vi "SS2 Live_Create HDF5 File.vi"(8 "error in (no error)":errorcluster, 11 "Current Data Set":i32) -> (0 "Error Out":errorcluster, 1 "Notebook Message":string, 2 "# Image Sets":u32, 3 "# Data Sets":i32, 5 "Data Q Name":string)   [LabVIEW 2019]
uses:
  SS2 Live_Settings List.ctl
  SS2 Live_File Information.ctl
  SS2 DAQ Parameters 2.ctl
  SS2 Gate Definition.ctl
  <vilib>/addons/h5labview2/file/H5Fmode.ctl
  <vilib>/Utility/error.llb/Error Cluster From Error Code.vi
  <vilib>/ErrorRing/Error Ring.xnode
  <vilib>/addons/h5labview2/file/H5F.lvlib
panel:
  out "File Folder":path
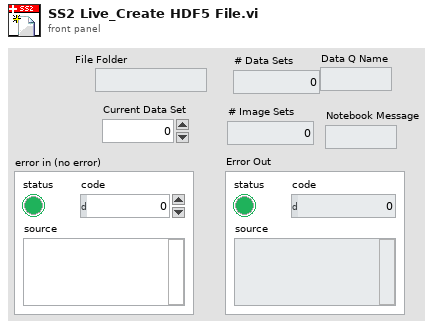
[diagram p1: front panel]
types:
  T1 = typedef "SS2 DAQ Parameters 2.ctl" = cluster{"10 bits":bool, "# Exposure Sequences":u32, "# 1-bit Frame per Gate":u32, "Gate Shift":u32, "# Gates per Set":u32, "# Sets":u32, "Laser Period":dbl[unit], "Gate Offset":u32, "Auto-adjust Gate Offset":bool, "Gate Definition":T2}
  T2 = typedef "SS2 Gate Definition.ctl" = cluster{"gs_psincdec_0":u32, "gs_psincdec_1":u32, "gs_psincdec_2":u32, "gs_psincdec_3":u32, "gs_no_shift_adj_1":u32, "gs_no_shift_adj_2":u32, "gs_no_shift_adj_3":u32}
  T3 = typedef "SS2 Live_Settings List.ctl" = enum16{"FPGA:Bitfile Path", "FPGA:Bitfile Version", "Acquisition Parameters:SS2 DAQ Parameters", "Acquisition Parameters:Gate Configuration Array", "Acquisition Parameters:Buffer Size (# Gates)", "File Information:File Information", "File Information:# Datasets in Series", "Image Parameters:Image ROI Information", "Image Parameters:Image Binning Options", "UI Parameters:Histogram Bins Number"}
  T4 = typedef "SS2 Live_File Information.ctl" = cluster{"File Folder":path, "File Name":string, "File Index":u32, "Author":string, "Sample":string, "Compression":bool}
  T5 = typedef "H5F.lvlib/H5Fmode.ctl" = enum16{"read-only", "read-write", "overwrite", "create new", "open or create"}
  T6 = typedef "hid_t.ctl" = i32
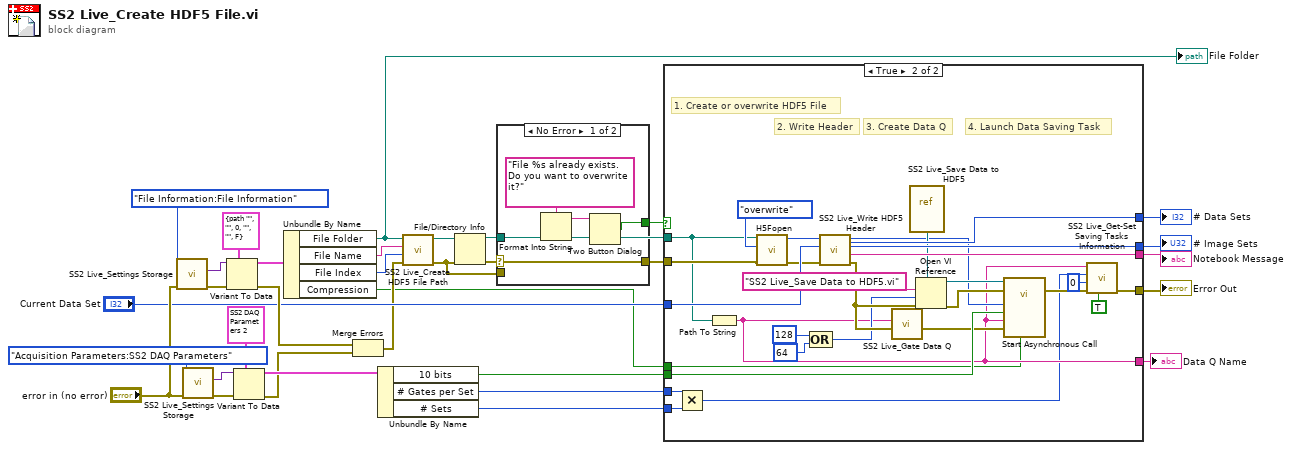
[diagram p0: block diagram]
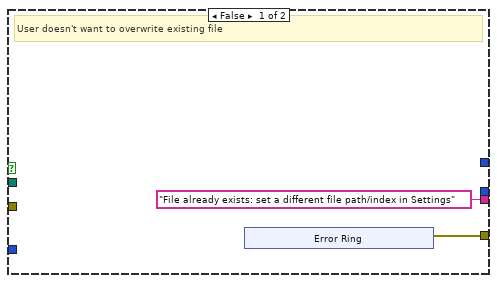
[diagram p2: hidden frame]
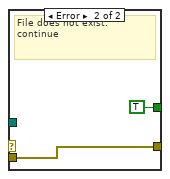
[diagram p3: hidden frame]
diagram:
  n1 = call "SS2 Live_Settings Storage.vi"("Error In"="error in (no error)", "Settings List"=SS2_Live_Settings_List."File Information:File Information") -> ("Error Out"=w32:errorcluster, "Variant Data out"=w31:variant)  [unwired: 8 in]
  n2 = call "SS2 Live_Settings Storage.vi"("Error In"="error in (no error)", "Settings List"=SS2_Live_Settings_List."Acquisition Parameters:SS2 DAQ Parameters") -> ("Error Out"=w23:errorcluster, "Variant Data out"=w22:variant)  [unwired: 8 in]
  n3 = Variant To Data(error in=w32, type=T4 {"File Folder"=path "", "File Name"="", "File Index"=0, "Author"="", "Sample"="", "Compression"=FALSE} ("File Information"), Variant=w31) -> (data=w29:T4, error out=w26:errorcluster)
  n4 = Variant To Data(error in=w23, type=T1 {"10 bits"=FALSE, "# Exposure Sequences"=0, "# 1-bit Frame per Gate"=0, "Gate Shift"=0, "# Gates per Set"=0, "# Sets"=1, "Laser Period"=0.0, "Gate Offset"=0, "Auto-adjust Gate Offset"=FALSE, "Gate Definition"={"gs_psincdec_0"=0, "gs_psincdec_1"=0, "gs_psincdec_2"=0, "gs_psincdec_3"=0, "gs_no_shift_adj_1"=0, "gs_no_shift_adj_2"=0, "gs_no_shift_adj_3"=0}} ("SS2 DAQ Parameters"), Variant=w22) -> (data=w20:T1, error out=w14:errorcluster)
  n5 = Unbundle By Name(w29) -> ("File Folder"=w28:path, "File Name"=w11:string, "File Index"=w27:u32, "Compression"=w1:bool)
  "File Folder" <- w28
  n6 = Merge Errors(w26, w14) -> (w15:errorcluster)
  n7 = Unbundle By Name(w20) -> ("10 bits"=w12:bool, "# Gates per Set"=w3:u32, "# Sets"=w2:u32)
  n8 = call "SS2 Live_Create HDF5 File Path.vi"("error in (no error)"=w15, "File Index"=w27, "File Name"=w11, "File Folder"=w28) -> ("error out"=w5:errorcluster, "File path"=w10:path)  [unwired: 6 in]
  n9 = File/Directory Info(path=w10, error in=w5) -> (path out=w8:path, error out=w9:errorcluster)  [unwired: 5 out]
  n10 = case shown="No Error" w9 {
    selector: w9 -> [w34 _]
    tunnel: w8 -> [w38 _]
    tunnel: [w35 TRUE ("T button?")] -> w7
    tunnel: [w34 w40] -> w6
    tunnel: w5 -> [_ w40]
    frame No Error {
      n11 = Format Into String(format string="File %s already exists. Do you want to overwrite it?", w38) -> (resulting string=w36:string)  [unwired: 2 in, 1 out]
      n12 = Two Button Dialog(message=w36) -> (T button?=w35:bool)  [unwired: 2 in]
    }
    frame Error {
      # "File does not exist:\ncontinue"
    }
  }
  n13 = case shown="True" w7 {
    tunnel: [_ w74] -> w19
    tunnel: ["File already exists: set a different file path/index in Settings" ("Notebook Message") w73] -> w18
    tunnel: [_ w71] -> w17
    tunnel: "Current Data Set" -> [_ w70]
    tunnel: [w41 w54] -> w13
    tunnel: w12 -> [_ w63]
    tunnel: w6 -> [_ w60]
    tunnel: w8 -> [_ w59]
    tunnel: [_ w53] -> w4
    tunnel: w3 -> [_ w52]
    tunnel: w2 -> [_ w51]
    tunnel: w1 -> [_ w47]
    frame False {
      # "User doesn't want to overwrite existing file"
      n14 = xnode "Error Ring"() -> ("error out"=w41:errorcluster)
    }
    frame True {
      # "4. Launch Data Saving Task"
      # "3. Create Data Q"
      # "2. Write Header"
      # "1. Create or overwrite HDF5 File"
      n15 = Multiply(x=w52, y=w51) -> (x*y=w50:u32)
      n16 = Path To String(path=w59) -> (string=w53:string)
      n17 = call <vilib>:"H5Fopen.vi"("error in (no error)"=w60, "mode (read-only)"=H5Fmode."overwrite", "path"=w59) -> ("error out"=w69:errorcluster, "ref out"=w72:T6)  [unwired: 7 in]
      n18 = Compound Arithmetic op=OR(128 ("options"), 64 ("options")) -> (w56:i32)
      n19 = call "SS2 Live_Write HDF5 Header.vi"("error in (no error)"=w69, "Current Data Set"=w70, "ref in"=w72) -> ("Error Out"=w62:errorcluster, "Notebook Message"=w73:string, "# Image Sets"=w74:u32, "ref out"=w64:T6, "# Data Sets"=w71:i32)  [unwired: 4 in]
      n20 = call "SS2 Live_Gate Data Q.vi"("error in (no error)"=w62, "SS2 Live Gate Data Q Name"=w53) -> ("error out"=w61:errorcluster)  [unwired: 4 in, 1 out]
      n21 = vi-ref "SS2 Live_Save Data to HDF5.vi"() -> (w67:refnum<vi>)
      n22 = Open VI Reference(type specifier VI Refnum (for type only)=w67, vi path="SS2 Live_Save Data to HDF5.vi" ("Notebook Message"), options=w56, error in (no error)=w62) -> (vi reference=w66:refnum<vi>, error out=w65:errorcluster)  [unwired: 2 in]
      n23 = call-by-ref "Start Asynchronous Call"(reference=w66, error in=w65, "Compression"=w47, 8:"error in (no error)"=w61, "SS2 Live Gate Data Q Name"=w53, "10-bit Gate Image"=w63, "HDF5 ref"=w64) -> (error out=w55:errorcluster)  [unwired: 6 in, 2 out]
      n24 = call "SS2 Live_Get-Set Saving Tasks Information.vi"("Get (F)/Set"=TRUE, "error in (no error)"=w55, "# New Images Saved (1)"=0 ("# New Images Saved"), "# Images (Total)"=w50, "File Path"=w53) -> ("error out"=w54:errorcluster)  [unwired: 3 in, 3 out]
    }
  }
  "Error Out" <- w13
  "# Image Sets" <- w19
  "Notebook Message" <- w18
  "# Data Sets" <- w17
  "Data Q Name" <- w4
